vi "serial_write_read.vi"(0 "VISA resource name":refnum<visa-resource-name>="COM7", 1 "baud rate":u32=115200, 2 "data bits":u16=8 min=5 max=8 step=1, 3 "parity":u16(ring) items=["None", "Odd", "Even", "Mark", "Space"], 4 "stop bits":u16(ring)=10 items=["1.0"=10, "1.5"=15, "2.0"=20], 6 "read":bool=TRUE, 7 "flow control":u16(ring) items=["None"=0, "XON/XOFF"=1, "RTS/CTS"=2, "DTR/DSR"=4]) -> (9 "read string":string, 10 "bytes read":u32)   [LabVIEW 2017]
doc: "The Basic Serial Read and Write example performs a Serial Port Read, a Serial Port Write, or a combination of these actions. The user selects the actions (read or write) on the front panel. If both are selected, the VI will write the data first, read data, and then close the VISA session that is opened to the port. This VI will wait until the specified number of bytes is received at the port. Only the number of bytes specified will be read.\n\nINSTRUCTIONS:\n1) Select the serial resource and configuration parameters (baud rate, data bits, parity, stop bits, flow control).\n2) Select the operations to be performed. \n3) Connect the serial port to your device. If no device is available, perform a loopback test by doing one of the following. Short pins 2 and 3 on a RS-232 cable or short pin 4 to pin 8 and pin 5 to pin 9 on a RS-485/422 cable. \n4) Run the VI to see the data read. (The \"read string\" will match the \"string to write\" if a loopback test was performed.)\n\nNote: The parameters set for the serial port must match the parameters of the connected instrument or device. In this example, the bytes to read parameter specifies the number of bytes that the serial port reads. If there were more bytes at the port than the number specified in bytes to read, those bytes would not be read. Also, if you specify to read more bytes than the number of bytes actually read, you might receive a timeout error message.\n\nOn the block diagram, the Configure Serial Port VI sets the configuration parameters. The front panel displays the controls used to configure the basic parameters, such as baud rate, data bits, and parity. Constants configure the other parameters the user probably does not need set. After the VISA Configure Serial Port VI opens the VISA session and configures the port, the VI passes the VISA resource name to other VIs that perform operations on that VISA resource. The VISA Write function sends a command to the serial device and the VISA Read function returns data based on the command. The VISA Close function then closes the reference to the serial device. It is important to close the reference; otherwise communication through with that port through protocols other than VISA might not be possible."
uses:
  <vilib>/Instr/_visa.llb/VISA Configure Serial Port (Instr).vi
panel:
  in  "wbc":dbl=4.0
  in  "Repeat":bool
  in  "delay before read (ms)":u32=500
  in  "string to write":string="ATZ\r\n"
  out "Return Count":u32
  in  "write":bool=TRUE
  in  "stop":bool
  # "Select the serial resource and the operations (Read, Write, or both) to be performed.  If both are selected, the VI will write the data first, read data and then close the VISA session that is opened to the port.  This VI will wait until the specified number of bytes is received at the port. Only the number of bytes specified will be read."
  # "For additional information select File >> VI Properties >> Documentation"
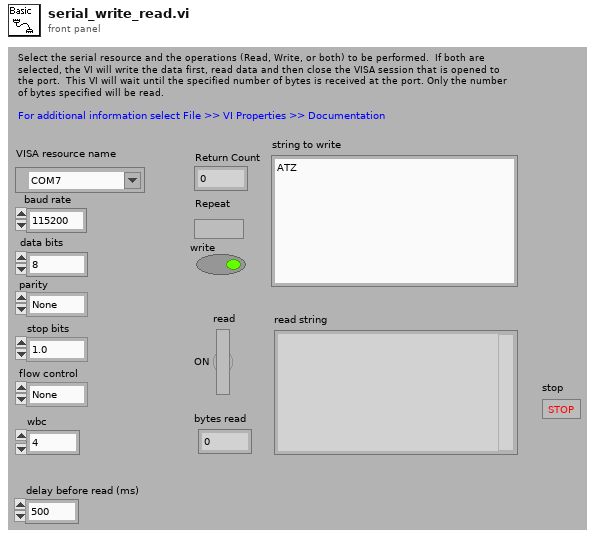
[diagram p1: front panel]
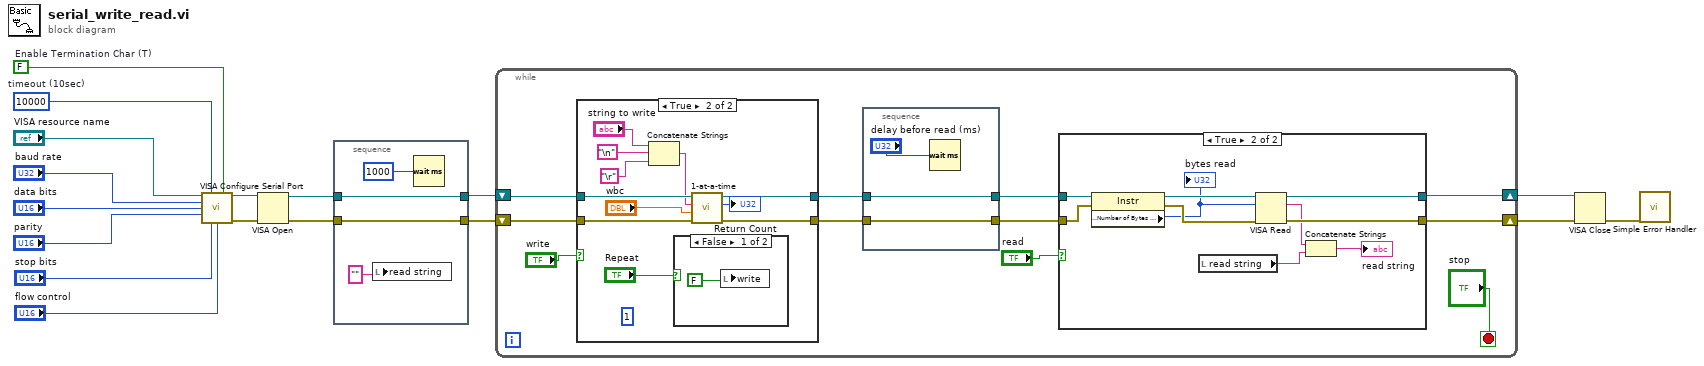
[diagram p0: block diagram]
diagram:
  w10 = FALSE  # Enable Termination Char (T)
  w11 = u32 10000  # timeout (10sec)
  n1 = call-poly "VISA Configure Serial Port"("VISA resource name"="VISA resource name", "timeout (10sec)"=w11, "Enable Termination\nChar (T)"=w10, "baud rate (9600)"="baud rate", "data bits (8)"="data bits", "parity (0:none)"="parity", "stop bits (10: 1 bit)"="stop bits", "flow control (0:none)"="flow control") -> ("VISA resource name out"=w6:refnum<visa-resource-name>, "error out"=w5:errorcluster)  [unwired: 6 in]
  n2 = VISA Open(error in (no error)=w5, VISA resource name=w6) -> (VISA resource name=w4:refnum<visa-resource-name>, error out=w3:errorcluster)  [unwired: 3 in]
  n3 = stacked-sequence {
    tunnel: w3 -> [w21]
    tunnel: [w21] -> w1
    tunnel: w4 -> [w20]
    tunnel: [w20] -> w2
    frame #0 {
      n4 = local write "read string"("") -> ()
      n5 = Wait (ms)(milliseconds to wait=u32 1000 ("delay before read (ms) 2")) -> ()  [unwired: 1 out]
    }
  }
  n6 = while {
    shift-right: [w31] -> w15
    shift-left: w1 -> [w24]
    shift-right: [w30] -> w14
    shift-left: w2 -> [w25]
    stop <- "stop" stop-if-true
    n7 = case shown="True" "write" {
      tunnel: [w37 w48] -> w27
      tunnel: w25 -> [w36 w47]
      tunnel: w24 -> [w37 w46]
      tunnel: [w36 w45] -> w26
      frame False {
      }
      frame True {
        (unwired) u32 1 ("Wait Between Characters(ms)")
        n8 = Concatenate Strings("string to write", "\n", "\r") -> (w42:string)
        n9 = case shown="False" "Repeat" {
          frame False {
            n10 = local write "write"(FALSE) -> ()
          }
          frame True {
          }
        }
        n11 = call "1-at-a-time.vi"("error in (no error)"=w46, "Wait Between Characters(ms)"="wbc", "write buffer"=w42, "VISA resource name"=w47) -> ("error out"=w48:errorcluster, "Return Count"=→"Return Count":u32, "VISA resource name out"=w45:refnum<visa-resource-name>)  [unwired: 5 in]
      }
    }
    n12 = stacked-sequence {
      tunnel: w27 -> [w35]
      tunnel: [w35] -> w22
      tunnel: w26 -> [w34]
      tunnel: [w34] -> w23
      frame #0 {
        n13 = Wait (ms)(milliseconds to wait="delay before read (ms)") -> ()  [unwired: 1 out]
      }
    }
    n14 = case shown="True" "read" {
      tunnel: w22 -> [w51 w57]
      tunnel: [w51 w61] -> w31
      tunnel: [w50 w60] -> w30
      tunnel: w23 -> [w50 w59]
      frame False {
      }
      frame True {
        n15 = property class="Instr"(reference=w59, error in=w57) -> (reference out=w58:refnum<visa-resource-name>, error out=w56:errorcluster, "Serial Settings:Number of Bytes at Serial Port"=w55:u32)
        "bytes read" <- w55
        n16 = local read "read string"() -> (w52:string)
        n17 = VISA Read(VISA resource name=w58, byte count=w55, error in (no error)=w56) -> (VISA resource name out=w60:refnum<visa-resource-name>, read buffer=w54:string, error out=w61:errorcluster)  [unwired: 1 out]
        n18 = Concatenate Strings(w54, w52) -> (→"read string":string)
      }
    }
  }
  n19 = VISA Close(VISA resource name=w14, error in (no error)=w15) -> (error out=w13:errorcluster)
  n20 = call <vilib>:"Simple Error Handler.vi"("error in (no error)"=w13) -> ()  [unwired: 4 in, 5 out]
